vi "NI PXIe-411x Rename channel.vi"(8 "error in (no error)":errorcluster, 11 "Node Ptr":T1 format="%.0x") -> (0 "error out":errorcluster, 3 "Node Ptr out":T1 format="%.0x")   [LabVIEW 2023, in "NI PXIe-411x PS Custom Device.lvlib"]
uses:
  NI PXIe-411x PS Custom Device.lvlib
  <vilib>/NI VeriStand/Custom Device API/Custom Device Item Ref.ctl
  411x_Global.vi
  <vilib>/NI VeriStand/Custom Device API/Get Item Property (U16).vi
  <vilib>/NI VeriStand/Custom Device API/Custom Device API.lvlib
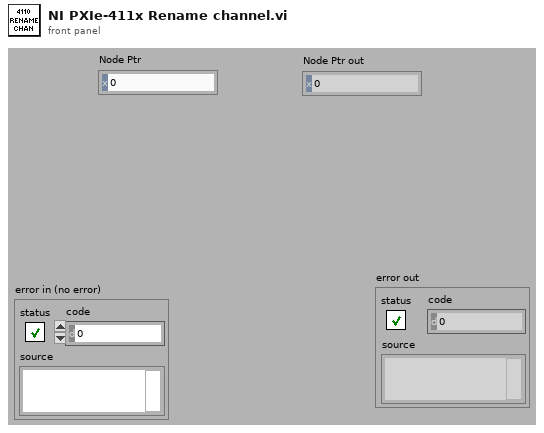
[diagram p1: front panel]
types:
  T1 = typedef "Custom Device API.lvlib/Custom Device Item Ref.ctl" = u64
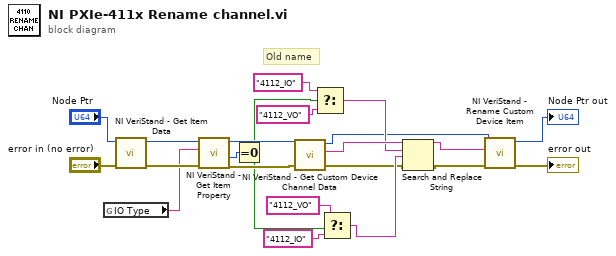
[diagram p0: block diagram]
diagram:
  # "Old name"
  n1 = global read "411x_Global.vi" "IO Type"() -> (w16:string)
  n2 = call <vilib>:"NI VeriStand - Get Item Data.vi"("error in (no error)"="error in (no error)", "Item Ref in"="Node Ptr") -> ("error out"=w17:errorcluster, "Item Ref out"=w18:T1)  [unwired: 8 out]
  n3 = call-poly <vilib>:"NI VeriStand - Get Item Property.vi"("error in (no error)"=w17, "Property Name"=w16, "Item Ref in"=w18) -> ("error out"=w12:errorcluster, "Value"=w13:u16, "Item Ref out"=w11:T1)  [unwired: 5 in, 1 out]
  n4 = Equal To 0?(x=w13) -> (x = 0?=w8:bool)
  n5 = call <vilib>:"NI VeriStand - Get Custom Device Channel Data.vi"("error in (no error)"=w12, "Channel Ref in"=w11) -> ("error out"=w2:errorcluster, "Channel Name"=w10:string, "Channel Ref out"=w3:T1)  [unwired: 4 in, 3 out]
  n6 = Select(t="4112_IO" ("string"), s=w8, f="4112_VO" ("string")) -> (s? t:f=w5:string)
  n7 = Select(t="4112_VO" ("string"), s=w8, f="4112_IO" ("string")) -> (s? t:f=w9:string)
  n8 = Search and Replace String(input string=w10, search string=w5, replace string=w9, error in=w2) -> (result string=w4:string, error out=w1:errorcluster)  [unwired: 4 in, 2 out]
  n9 = call <vilib>:"NI VeriStand - Rename Custom Device Item.vi"("error in (no error)"=w1, "New Name"=w4, "Item Ref in"=w3) -> ("error out"=→"error out":errorcluster, "Item Ref out"=→"Node Ptr out":T1)  [unwired: 1 in, 6 out]
